vi "FFT PtByPt.vi"   [LabVIEW 2017, in "NI_PtbyPt.lvlib"]
doc: "Computes the Fourier transform of <B>x</B>. This VI is similar to the FFT VI. Wire data to the <B>x</B> input to determine the polymorphic instance to use or manually select the instance."
uses:
  <vilib>/ptbypt/NI_PtbyPt.lvlib
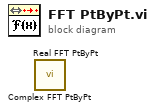
[diagram p0: block diagram]
diagram:
  n1 = call <vilib>:"Complex FFT PtByPt.vi"() -> ()  [unwired: 4 in, 2 out]
  n2 = call <vilib>:"Real FFT PtByPt.vi"() -> ()  [unwired: 4 in, 2 out]
